vi "Set discriminator.vi"(8 "error in (no error)":errorcluster, 9 "j (0)":T1, 10 "i (0)":T2, 11 "VISA resource name":refnum<visa-resource-name>) -> (0 "error out":errorcluster, 3 "VISA resource name out":refnum<visa-resource-name>)   [LabVIEW 2015, in "SR400.lvlib"]
doc: "DM i { ,j }\nThe DM command sets and reads the\ndiscriminator modes. i = 0,1, or 2 designates\ndiscriminator A,B, or T and is required. If j is\nincluded, the selected discriminator is set to\nFIXED, j=0, or SCAN, j=1. If j is absent, the\nmode of discriminator i is returned. The mode may\nbe changed during a scan. If it is changed to\nSCAN, the level begins scanning from the start\nvalue on the next count period. If it is changed to\nFIXED, the level returns to the start value\nimmediately."
uses:
  SR400.lvlib
  Typedefs/Counter.ctl
  Typedefs/Discriminator Output.ctl
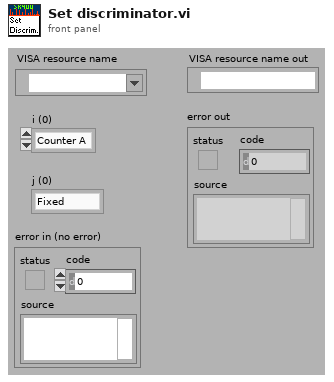
[diagram p1: front panel]
types:
  T1 = typedef "SR400.lvlib/Discriminator Output.ctl" = enum16{"Fixed", "Scan"}
  T2 = typedef "SR400.lvlib/Counter.ctl" = enum16{"Counter A", "Counter B", "Counter T"}
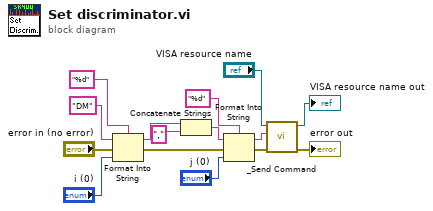
[diagram p0: block diagram]
diagram:
  n1 = Format Into String(format string="%d", initial string="DM" ("command"), error in="error in (no error)", "i (0)") -> (resulting string=w12:string, error out=w13:errorcluster)
  n2 = Concatenate Strings(w12, "," ("command")) -> (w7:string)
  n3 = Format Into String(format string="%d", initial string=w7, error in=w13, "j (0)") -> (resulting string=w4:string, error out=w3:errorcluster)
  n4 = call "_Send Command.vi"("error in (no error)"=w3, "Command"=w4, "VISA resource name"="VISA resource name") -> ("error out"=→"error out":errorcluster, "VISA resource name out"=→"VISA resource name out":refnum<visa-resource-name>)  [unwired: 1 in, 6 out]
